vi "Queued State Machine with UI Event Handling.vi"() -> ()   [LabVIEW 2009]
doc: "Ce VI est un modèle de machine à états basée sur une file d'attente. Remplacez Processus 1 et Processus 2 par vos états. Pour ajouter d'autres processus, modifiez la constante énumération à définition de type. L'ordre de l'énumération doit correspondre à celui du cluster."
uses:
  State Enum.ctl
panel:
  in  "stop":bool
  in  "Processus 2":bool
  in  "Processus 1":bool
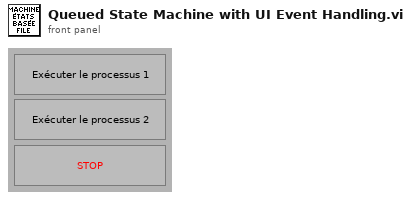
[diagram p1: front panel]
types:
  T1 = typedef "State Enum.ctl" = enum32{"Attente d'événements", "Processus 1", "Processus 2", "Arrêt"}
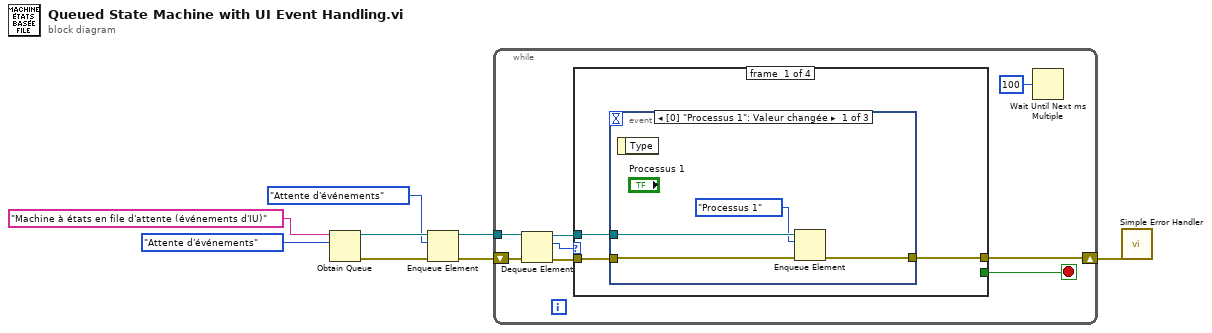
[diagram p0: block diagram]
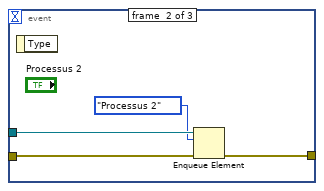
[diagram p2: hidden frame]
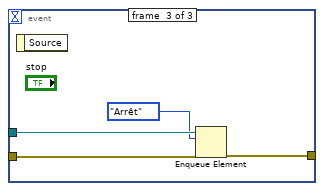
[diagram p3: hidden frame]
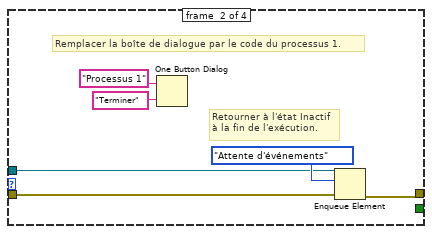
[diagram p4: hidden frame]
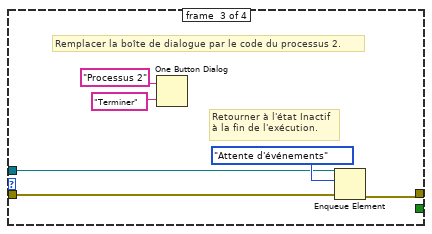
[diagram p5: hidden frame]
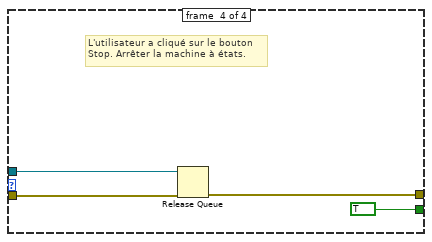
[diagram p6: hidden frame]
diagram:
  n1 = Obtain Queue ("Obtenir une file d'attente")(name (unnamed)="Machine à états en file d'attente (événements d'IU)", element data type=State_Enum."Attente d'événements" ("Enum")) -> (queue out=w6:refnum<queue>, error out=w7:errorcluster)  [unwired: 3 in, 1 out]
  n2 = Enqueue Element ("Ajouter un élément à la fin d'une file d'attente")(queue=w6, element=State_Enum."Attente d'événements" ("Enum"), error in (no error)=w7) -> (queue out=w4:refnum<queue>, error out=w5:errorcluster)  [unwired: 2 out]
  n3 = while "Boucle While" {
    tunnel: w4 -> [w11]
    shift-right: [w14] -> w1
    shift-left: w5 -> [w13]
    stop <- w16 stop-if-true
    n4 = Dequeue Element ("Supprimer le premier élément d'une file d'attente")(queue=w11, error in (no error)=w13) -> (queue out=w10:refnum<queue>, element=w9:T1, error out=w12:errorcluster)  [unwired: 2 out]
    n5 = case "Structure Condition" shown="\"Attente d'événements\", Par défaut" w9 {
      tunnel: [_ _ _ TRUE] -> w16
      tunnel: w12 -> [w18 w35 w41 w46]
      tunnel: w10 -> [w19 w32 w38 w45]
      tunnel: [w17 w34 w40 w44] -> w14
      frame #0 {
        n6 = event shown="[0] \"Processus 1\": Valeur changée" {
          selector: _ -> [_ _ _]
          dyn-events: _ -> [_ _ _]
          timeout: _ -> [_ _ _]
          tunnel: w19 -> [w23 w27 w31]
          tunnel: w18 -> [w22 w26 w30]
          tunnel: [w21 w25 w29] -> w17
          event #0 {
            n7 = event-data() -> ()  [unwired: 2 out]
            n8 = Enqueue Element(queue=w23, element=State_Enum."Processus 1" ("Enum"), error in (no error)=w22) -> (error out=w21:errorcluster)  [unwired: 1 in, 2 out]
          }
          event #1 {
            n9 = event-data() -> ()  [unwired: 2 out]
            n10 = Enqueue Element(queue=w27, element=State_Enum."Processus 2" ("Enum"), error in (no error)=w26) -> (error out=w25:errorcluster)  [unwired: 1 in, 2 out]
          }
          event #2 {
            n11 = event-data() -> ()  [unwired: 2 out]
            n12 = Enqueue Element(queue=w31, element=State_Enum."Arrêt" ("Enum"), error in (no error)=w30) -> (error out=w29:errorcluster)  [unwired: 1 in, 2 out]
          }
        }
      }
      frame #1 {
        # "Retourner à l'état Inactif\nà la fin de l'exécution."
        # "Remplacer la boîte de dialogue par le code du processus 1."
        n13 = One Button Dialog(message="Processus 1", button name ("OK")="Terminer") -> ()  [unwired: 1 out]
        n14 = Enqueue Element(queue=w32, element=State_Enum."Attente d'événements" ("Enum"), error in (no error)=w35) -> (error out=w34:errorcluster)  [unwired: 3 out]
      }
      frame #2 {
        # "Retourner à l'état Inactif\nà la fin de l'exécution."
        # "Remplacer la boîte de dialogue par le code du processus 2."
        n15 = One Button Dialog(message="Processus 2", button name ("OK")="Terminer") -> ()  [unwired: 1 out]
        n16 = Enqueue Element(queue=w38, element=State_Enum."Attente d'événements" ("Enum"), error in (no error)=w41) -> (error out=w40:errorcluster)  [unwired: 3 out]
      }
      frame #3 {
        # "L'utilisateur a cliqué sur le bouton\nStop. Arrêter la machine à états."
        n17 = Release Queue(queue=w45, error in (no error)=w46) -> (error out=w44:errorcluster)  [unwired: 1 in, 2 out]
      }
    }
    n18 = Wait Until Next ms Multiple ("Attendre un multiple de ms")(millisecond multiple=u32 100) -> ()  [unwired: 1 out]
  }
  n19 = call <vilib>:"Simple Error Handler.vi"("error in (no error)"=w1) -> ()  [unwired: 1 in, 8 out]
